vi "Write configuration.vi"(8 "error in":errorcluster, 10 "configuration":refnum<class "NISE_CEF_serializable configuration.lvclass">, 11 "Standard Engine Editor Node in":refnum<class "Standard Engine Editor Node.lvclass">) -> (0 "error out":errorcluster, 3 "Standard Engine Editor Node out":refnum<class "Standard Engine Editor Node.lvclass">)   [LabVIEW 2013, in "Standard Engine Editor Node.lvclass"]
uses:
  Standard Engine Editor Node.lvclass
  <vilib>/NI/Configuration Framework/serializable configuration/NISE_CEF_serializable configuration.lvclass
  Execution Engine/Configuration/Standard Engine Configuration.lvclass
  Standard Engine Editor Node.lvclass/Standard Engine Editor Node.ctl
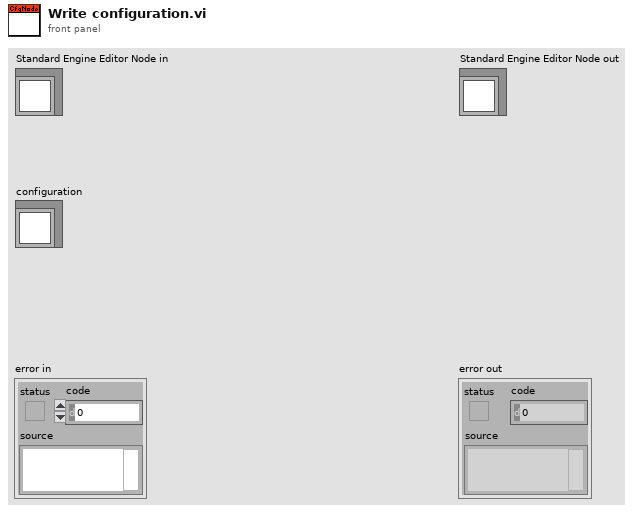
[diagram p1: front panel]
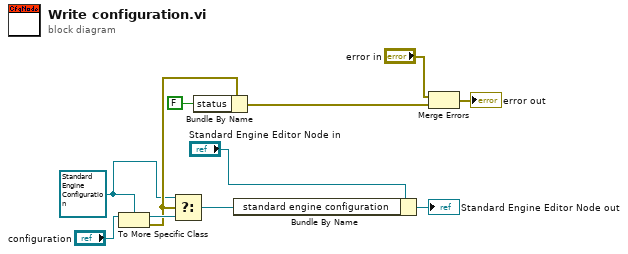
[diagram p0: block diagram]
diagram:
  w5 = refnum<class "Standard Engine Configuration.lvclass"> refnum ("standard engine configuration")
  n1 = To More Specific Class(target class=w5, reference="configuration") -> (specific class reference=w11:refnum<class "Standard Engine Configuration.lvclass">, error out=w10:errorcluster)  [unwired: 1 in]
  n2 = Select(t=w5, s=w10, f=w11) -> (s? t:f=w7:refnum<class "Standard Engine Configuration.lvclass">)
  n3 = Bundle By Name(cluster=w10, "status"=FALSE) -> (w8:errorcluster)
  n4 = Bundle By Name(cluster="Standard Engine Editor Node in", "standard engine configuration"=w7) -> (→"Standard Engine Editor Node out":refnum<class "Standard Engine Editor Node.lvclass">)
  n5 = Merge Errors("error in", w8) -> (→"error out":errorcluster)
